vi "eval_length_based.vi"(8 "error in (no error)":errorcluster, 9 "Min":i32, 10 "Max":i32, 11 "SN":string) -> (0 "error out":errorcluster, 1 "Device Type out":T1, 2 "SN ok?":bool, 3 "SN out":string)   [LabVIEW 2024]
uses:
  controls/SN_device_type_out.ctl
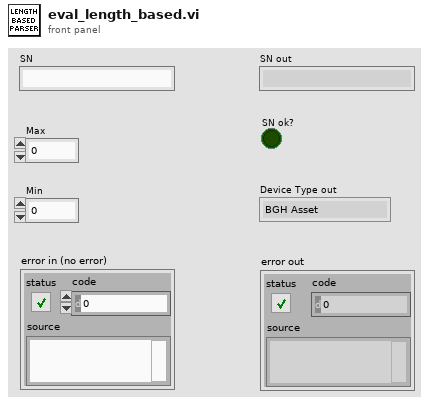
[diagram p1: front panel]
types:
  T1 = typedef "SN_device_type_out.ctl" = enum16{"BGH Asset", "BGH Product", "SAMSUNG Product", "GENERIC Product", "No Product", ""}
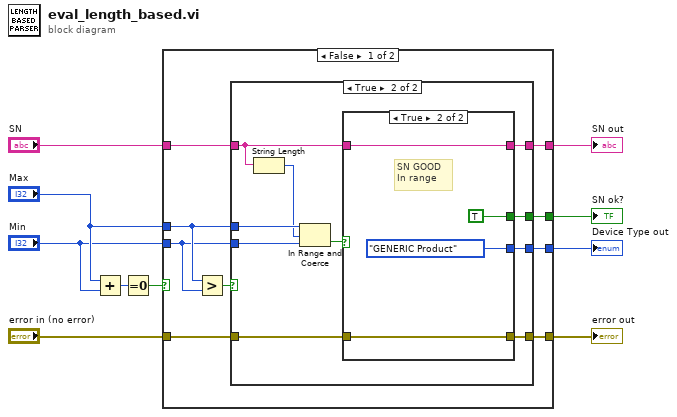
[diagram p0: block diagram]
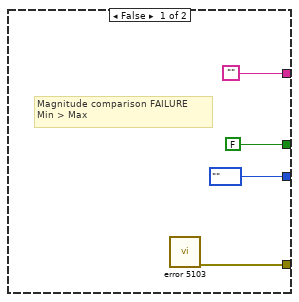
[diagram p2: hidden frame]
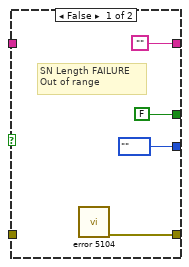
[diagram p3: hidden frame]
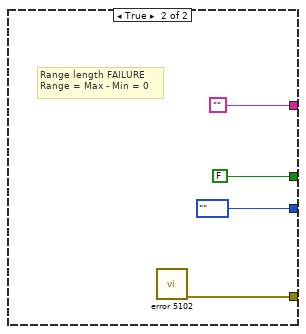
[diagram p4: hidden frame]
diagram:
  n1 = Add(x="Max", y="Min") -> (x+y=w4:i32)
  n2 = Equal To 0?(x=w4) -> (x = 0?=w5:bool)
  n3 = case shown="False" w5 {
    tunnel: [w18 w45] -> w6
    tunnel: "error in (no error)" -> [w17 _]
    tunnel: "Max" -> [w15 _]
    tunnel: "Min" -> [w14 _]
    tunnel: "SN" -> [w16 _]
    tunnel: [w13 SN_device_type_out."" ("Device Type out")] -> w3
    tunnel: [w12 FALSE] -> w2
    tunnel: [w11 ""] -> w1
    frame False {
      n4 = Greater?(x=w15, y=w14) -> (0:w19:bool)
      n5 = case shown="True" w19 {
        tunnel: [w23 w27] -> w18
        tunnel: w17 -> [_ w26]
        tunnel: w16 -> [_ w25]
        tunnel: w15 -> [_ w33]
        tunnel: w14 -> [_ w32]
        tunnel: [SN_device_type_out."" ("Device Type out") w29] -> w13
        tunnel: [FALSE w28] -> w12
        tunnel: ["" w24] -> w11
        frame False {
          # "Magnitude comparison FAILURE\nMin > Max"
          n6 = call "error 5103.vi"() -> ("error out"=w23:errorcluster)  [unwired: 11 in]
        }
        frame True {
          n7 = String Length(string=w25) -> (length=w31:i32)
          n8 = In Range and Coerce(upper limit=w33, x=w31, lower limit=w32) -> (In Range?=w30:bool)  [unwired: 1 out]
          n9 = case shown="True" w30 {
            tunnel: [SN_device_type_out."" ("Device Type out") SN_device_type_out."GENERIC Product" ("Device Type out")] -> w29
            tunnel: [FALSE TRUE] -> w28
            tunnel: [w35 w39] -> w27
            tunnel: w26 -> [_ w39]
            tunnel: w25 -> [_ w38]
            tunnel: ["" w38] -> w24
            frame False {
              # "SN Length FAILURE\nOut of range"
              n10 = call "error 5104.vi"() -> ("error out"=w35:errorcluster)  [unwired: 11 in]
            }
            frame True {
              # "SN GOOD\nIn range"
            }
          }
        }
      }
    }
    frame True {
      # "Range length FAILURE\nRange = Max - Min = 0"
      n11 = call "error 5102.vi"() -> ("error out"=w45:errorcluster)  [unwired: 11 in]
    }
  }
  "error out" <- w6
  "Device Type out" <- w3
  "SN ok?" <- w2
  "SN out" <- w1
